vi "configure image.vi"(9 "Number of B-scan":i32, 10 "Number of records":i32, 11 "Zoom Factor":sgl) -> (3 "Draw Area Size":T1)   [LabVIEW 2014]
uses:
  <vilib>/Utility/miscctls.llb/LVBoundsTypeDef.ctl
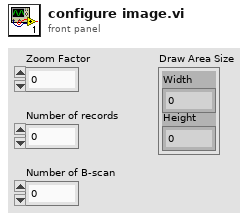
[diagram p1: front panel]
types:
  T1 = typedef "LVBoundsTypeDef.ctl" = cluster{"Width":u32, "Height":u32}
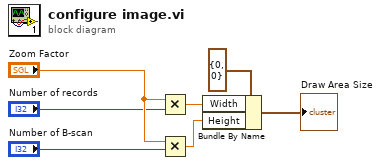
[diagram p0: block diagram]
diagram:
  n1 = Multiply(x="Zoom Factor", y="Number of records") -> (x*y=w3:sgl)
  n2 = Multiply(x="Zoom Factor", y="Number of B-scan") -> (x*y=w5:sgl)
  n3 = Bundle By Name(cluster=T1 {"Width"=0, "Height"=0} ("Draw Area Size"), "Width"=w3, "Height"=w5) -> (→"Draw Area Size":T1)
